vi "storeRobotModelTestCrashCases.vi"(5 "est_vel":dbl format="%#_13g", 7 "CrashCases":T1[](array[typedef]), 8 "error in (no error)":errorcluster, 9 "RealVelocities":dbl[][](array[numeric]), 10 "IdealVelocities":dbl[][](array[numeric]), 11 "Game in":refnum<class "Game.lvclass">) -> (0 "error out":errorcluster, 2 "CrashCasesArray out":T1[](array[typedef]), 3 "Game out":refnum<class "Game.lvclass">)   [LabVIEW 2021, in "Game.lvclass"]
uses:
  Game.lvclass
  Controls/RobotModelTestCrashCase.ctl
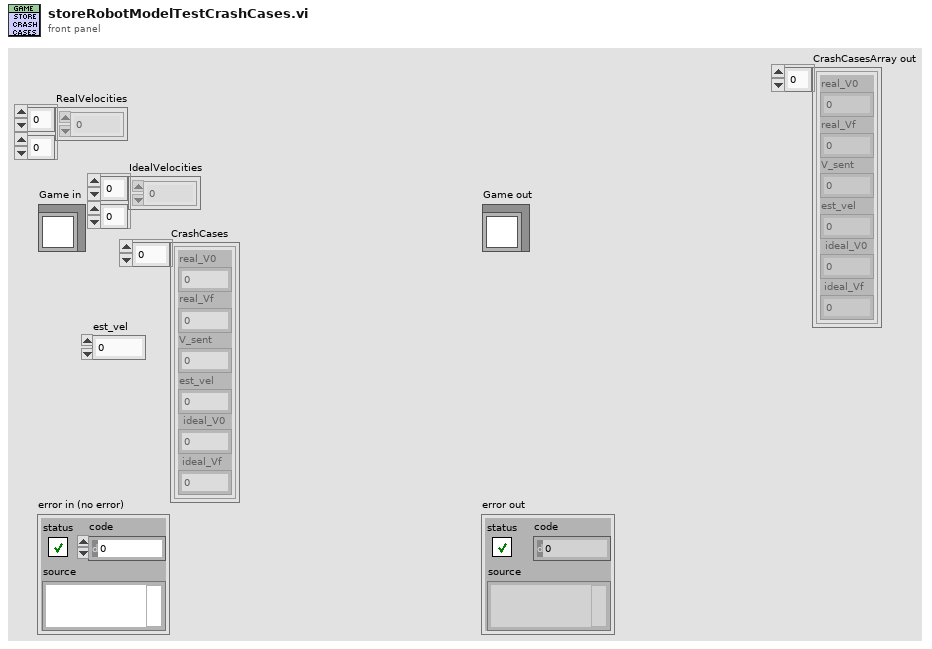
[diagram p1: front panel]
types:
  T1 = typedef "RobotModelTestCrashCase.ctl" = cluster{"real_V0":dbl, "real_Vf":dbl, "V_sent":dbl, "est_vel":dbl, "ideal_V0":dbl, "ideal_Vf":dbl}
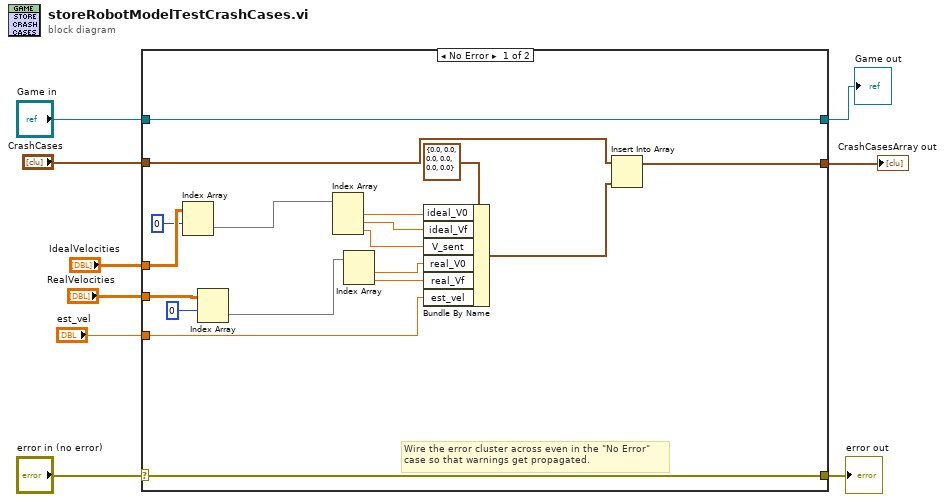
[diagram p0: block diagram]
diagram:
  n1 = case shown="No Error" "error in (no error)" {
    selector: "error in (no error)" -> [w26 w29]
    tunnel: [w26 w29] -> w8
    tunnel: [w27 w28] -> w6
    tunnel: "Game in" -> [w27 w28]
    tunnel: "CrashCases" -> [w11 _]
    tunnel: "est_vel" -> [w10 _]
    tunnel: [w24 _] -> w4
    tunnel: "IdealVelocities" -> [w23 _]
    tunnel: "RealVelocities" -> [w16 _]
    frame No Error {
      # "Wire the error cluster across even in the \"No Error\"\ncase so that warnings get propagated."
      n2 = Index Array(array=w23, index (row)=0) -> (element=w21:dbl[])  [unwired: 1 in]
      n3 = Index Array(array=w16, index (row)=0) -> (element=w15:dbl[])  [unwired: 1 in]
      n4 = Index Array(array=w21) -> (element #1=w20:dbl, element #2=w19:dbl, element #3=w18:dbl)  [unwired: 3 in]
      n5 = Index Array(array=w15) -> (element #1=w14:dbl, element #2=w13:dbl)  [unwired: 2 in]
      n6 = Bundle By Name(cluster=T1 {"real_V0"=0.0, "real_Vf"=0.0, "V_sent"=0.0, "est_vel"=0.0, "ideal_V0"=0.0, "ideal_Vf"=0.0} ("CrashCases 2"), "ideal_V0"=w20, "ideal_Vf"=w19, "V_sent"=w18, "real_V0"=w14, "real_Vf"=w13, "est_vel"=w10) -> (w25:T1)
      n7 = Insert Into Array(array=w11, new element=w25) -> (w24:T1[])  [unwired: 1 in]
    }
    frame Error {
    }
  }
  "error out" <- w8
  "Game out" <- w6
  "CrashCasesArray out" <- w4
